vi "Waveforms.vi"() -> ()   [LabVIEW 2020]
panel:
  out "Phase (°)":dbl
  in  "Phase (°)":dbl(knob) scale=0.0..360.0
  out "Duty Cycle (%)":dbl
  out "Frequency (Hz)":dbl
  out "Amplitude (V)":dbl
  in  "Duty Cycle (%)":dbl(knob) scale=0.0..100.0
  in  "Wave selector":string(combo)
  in  "Frequency (Hz)":dbl(knob) scale=1.0..500.0
  in  "Amplitude (V)":dbl(knob) scale=0.0..200.0
  out "Waveform Graph":dynamicdata(graph)
  in  "stop":bool
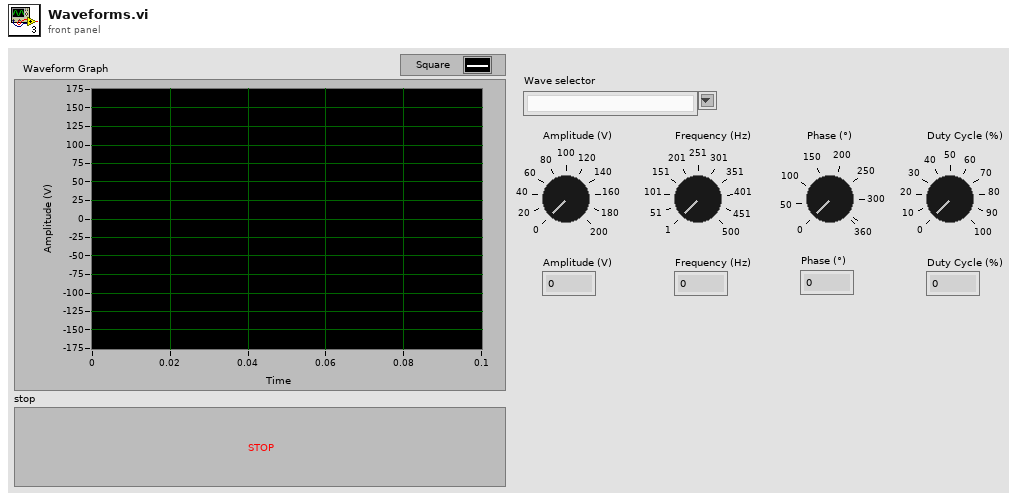
[diagram p1: front panel]
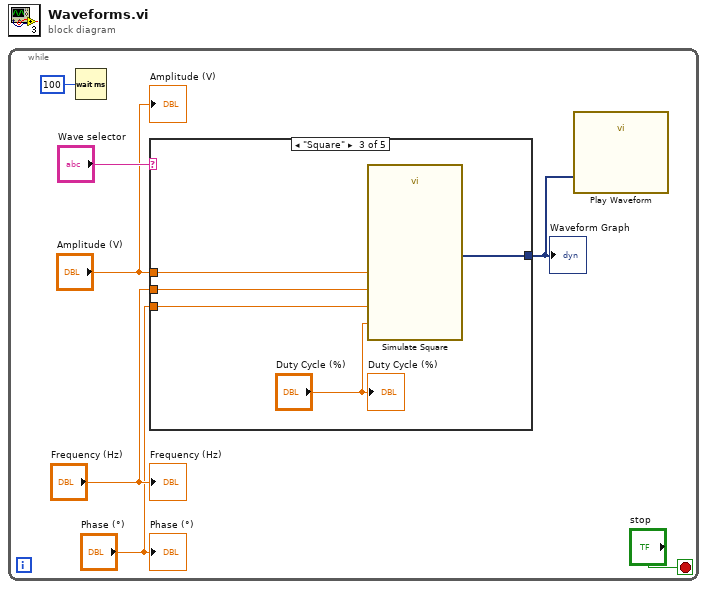
[diagram p0: block diagram]
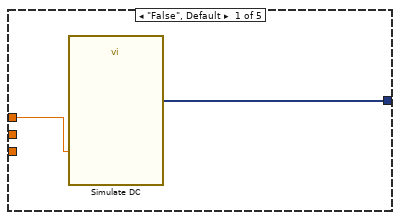
[diagram p2: hidden frame]
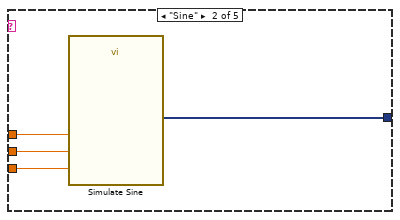
[diagram p3: hidden frame]
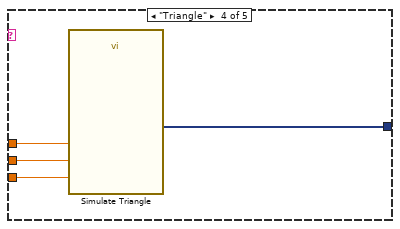
[diagram p4: hidden frame]
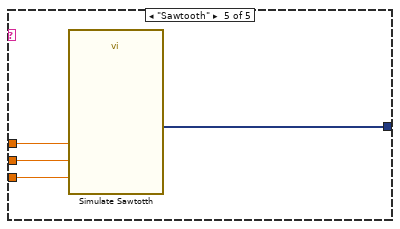
[diagram p5: hidden frame]
diagram:
  n1 = while {
    stop <- "stop" stop-if-true
    n2 = Wait (ms)(milliseconds to wait=u32 100) -> ()  [unwired: 1 out]
    n3 = case shown="\"Square\"" "Wave selector" {
      tunnel: "Frequency (Hz)" -> [_ w13 w18 w22 w26]
      tunnel: "Amplitude (V)" -> [w8 w12 w17 w21 w25]
      tunnel: [w9 w10 w14 w19 w23] -> w1
      tunnel: "Phase (°)" -> [_ w11 w15 w20 w24]
      frame "False", Default {
        n4 = call "Simulate DC"("Offset"=w8) -> ("DC"=w9:dynamicdata)  [unwired: 13 in, 1 out]
      }
      frame "Sine" {
        n5 = call "Simulate Sine"("Frequency"=w13, "Amplitude"=w12, "Phase"=w11) -> ("Sine"=w10:dynamicdata)  [unwired: 11 in, 1 out]
      }
      frame "Square" {
        n6 = call "Simulate Square"("Duty Cycle (%)"="Duty Cycle (%)", "Frequency"=w18, "Amplitude"=w17, "Phase"=w15) -> ("Square"=w14:dynamicdata)  [unwired: 10 in, 1 out]
        "Duty Cycle (%)" <- "Duty Cycle (%)"
      }
      frame "Triangle" {
        n7 = call "Simulate Triangle"("Frequency"=w22, "Amplitude"=w21, "Phase"=w20) -> ("Triangle"=w19:dynamicdata)  [unwired: 11 in, 1 out]
      }
      frame "Sawtooth" {
        n8 = call "Simulate Sawtotth"("Frequency"=w26, "Amplitude"=w25, "Phase"=w24) -> ("Sawtooth"=w23:dynamicdata)  [unwired: 11 in, 1 out]
      }
    }
    "Waveform Graph" <- w1
    n9 = call "Play Waveform"("Data"=w1) -> ()  [unwired: 18 in, 1 out]
    "Amplitude (V)" <- "Amplitude (V)"
    "Frequency (Hz)" <- "Frequency (Hz)"
    "Phase (°)" <- "Phase (°)"
  }
